vi "LVUSBRH2_Measurement_main.vi"() -> ()   [LabVIEW 2020]
uses:
  <vilib>/Utility/sysdir.llb/System Directory Type.ctl
  <vilib>/Utility/miscctls.llb/LVPointTypeDef.ctl
  <vilib>/Instr/_visa.llb/VISA Flush IO Buffer Mask.ctl
  <vilib>/Platform/browser.llb/Open URL in Default Browser (string).vi
  <vilib>/Instr/_visa.llb/VISA Configure Serial Port (Instr).vi
  <vilib>/ptbypt/NI_PtbyPt.lvlib
panel:
  in  "USBRH Link":bool caption="USBRRH2 link:"
  out "title":string="LVUSBRH2 Measure"
  out "Measure":bool
  in  "Btn Exit":bool
  in  "LED 2":bool
  in  "LED 1":bool
  in  "Btn Settings":bool
  in  "Btn Stop":bool
  in  "Btn Start":bool
  out "Humid":dbl caption="RHumidity(%)" format="%.2f"
  out "Temp":dbl caption="Temperature(C)" format="%.2f"
  out "chart 1":cluster{dbl, dbl}(graph)
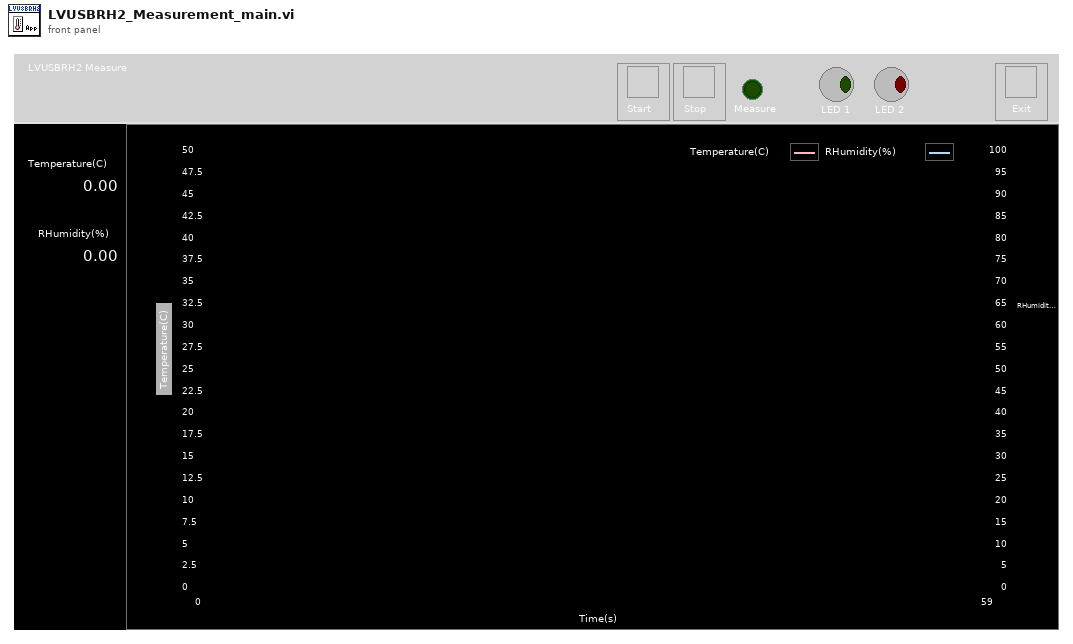
[diagram p1: front panel]
types:
  T1 = typedef "System Directory Type.ctl" = i32
  T2 = typedef "LVPointTypeDef.ctl" = cluster{"Horizontal":i16, "Vertical":i16}
  T3 = cluster{bool, "include Ctrl key?":bool, string}[]
  T4 = cluster{"配列[0]":i16, "配列[1]":i16, "配列[2]":i16, "配列[3]":i16}
  T5 = typedef "VISA Flush IO Buffer Mask.ctl" = u16
  T6 = typedef "LVRectTypeDef.ctl" = cluster{"left":i16, "top":i16, "right":i16, "bottom":i16}
  T7 = enum32{"invalid app kind", "Development System", "Run Time System", "Student Edition", "Embedded LabVIEW", "Evaluation", "Custom"}
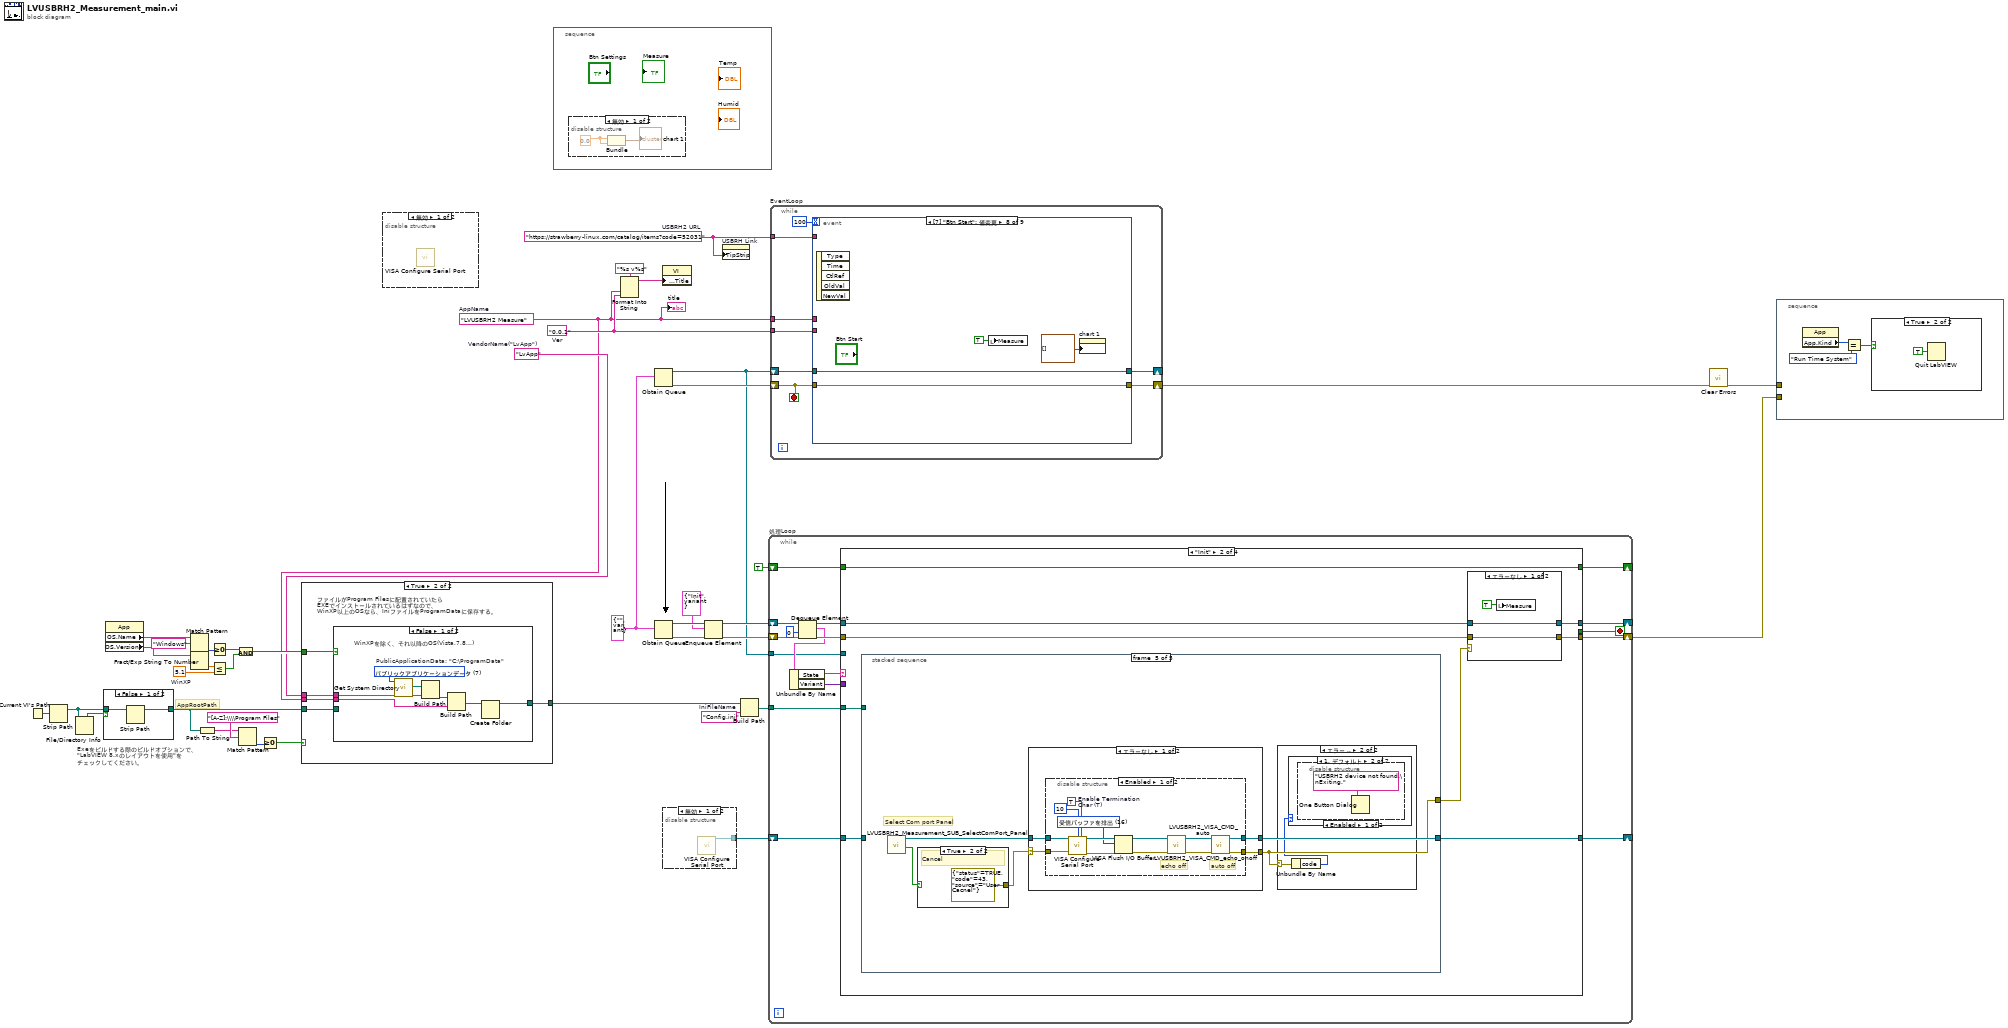
[diagram p0: block diagram]
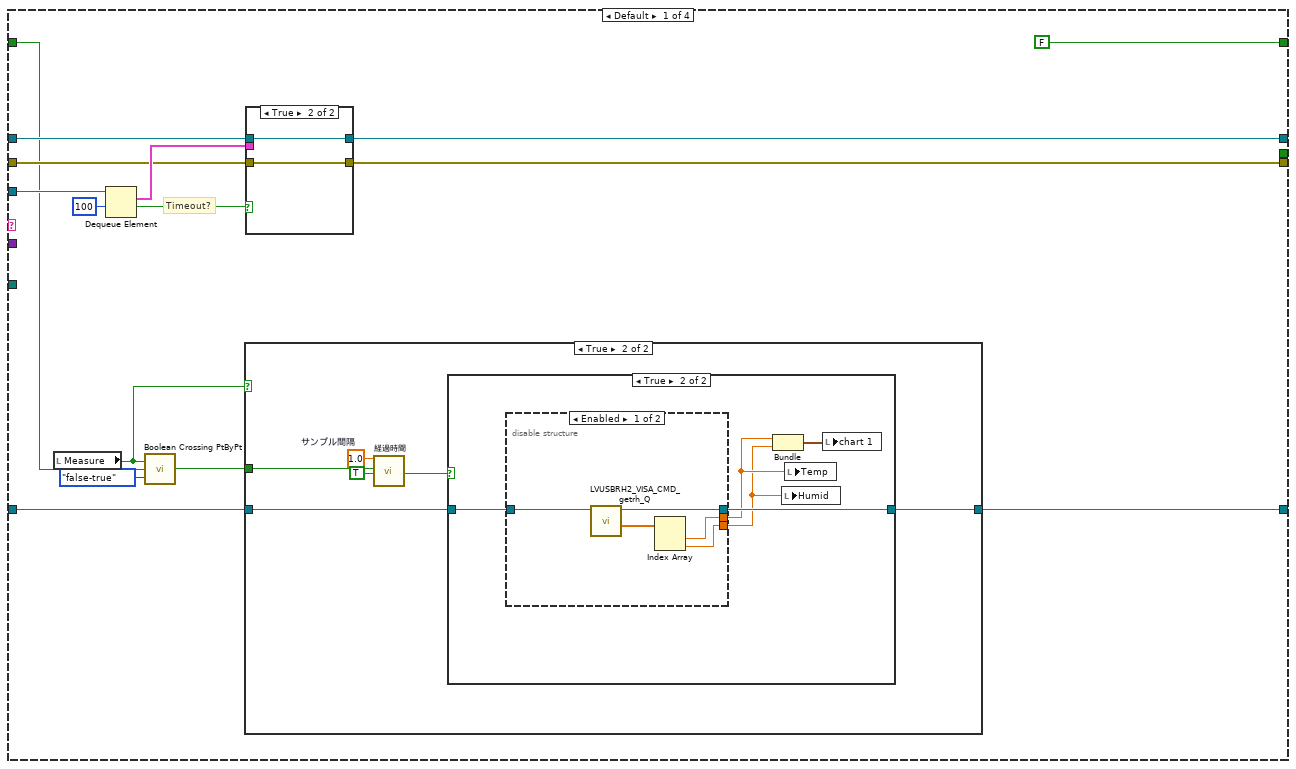
[diagram p9: hidden frame]
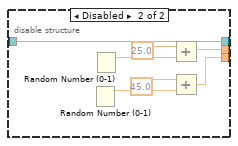
[diagram p12: hidden frame]
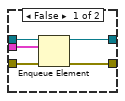
[diagram p13: hidden frame]
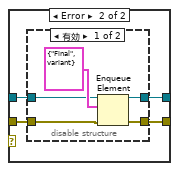
[diagram p14: hidden frame]
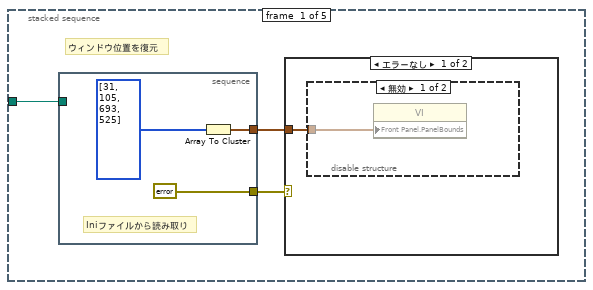
[diagram p16: hidden frame]
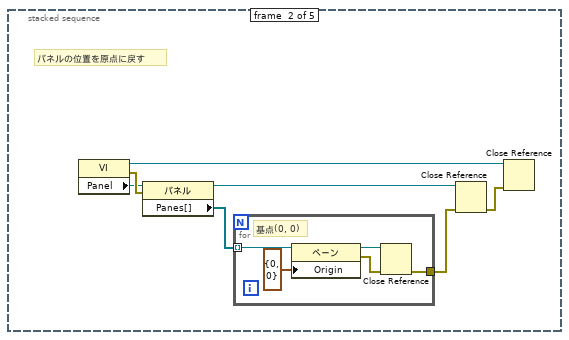
[diagram p19: hidden frame]
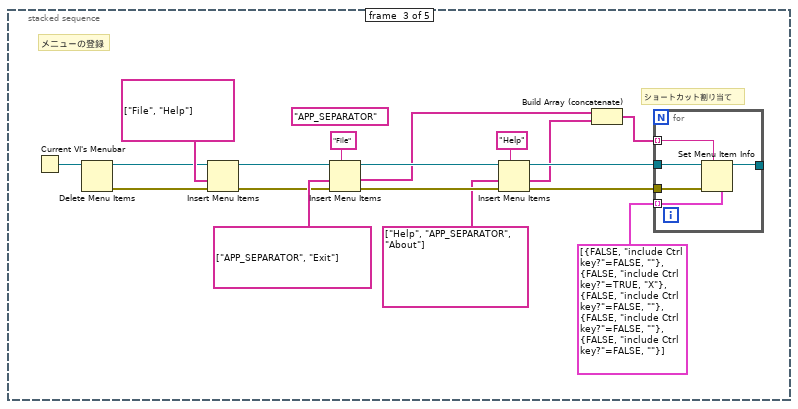
[diagram p20: hidden frame]
diagram:
  w3 = "LvApp"  # VendorName("LvApp")
  w17 = 5.1  # WinXP
  w23 = "https://strawberry-linux.com/catalog/items?code=52031"  # USBRH2 URL
  w25 = "Config.ini"  # IniFileName
  w28 = "0.0.1"  # Ver
  w2 = "LVUSBRH2 Measure"  # AppName
  w39 = cluster{"State":string, "Variant":variant} {"State"="", "Variant"=variant}
  # "Exeをビルドする際のビルドオプションで、\n\"LabVIEW 8.xのレイアウトを使用\"を\nチェックしてください。"
  # "AppRootPath"
  n1 = Current VI's Path() -> (path=w11:path)
  n2 = Strip Path(path=w11) -> (stripped path=w12:path)  [unwired: 1 out]
  n3 = File/Directory Info(path=w12) -> (directory=w13:bool)  [unwired: 1 in, 6 out]
  n4 = case shown="FALSE" w13 {
    tunnel: w12 -> [w41 w42]
    tunnel: [w40 w42] -> w8
    frame False {
      n5 = Strip Path(path=w41) -> (stripped path=w40:path)  [unwired: 1 out]
    }
    frame True {
    }
  }
  n6 = property class="App"() -> ("OS.Name"=w21:string, "OS.Version"=w19:string)  [unwired: 2 in, 2 out]
  n7 = Match Pattern(string=w21, regular expression="Windows" ("正規表現")) -> (offset past match=w16:i32)  [unwired: 1 in, 3 out]
  n8 = Fract/Exp String To Number(string=w19) -> (number=w18:dbl)  [unwired: 3 in, 1 out]
  n9 = Path To String(path=w8) -> (string=w7:string)
  n10 = Greater Or Equal To 0?(x=w16) -> (x >= 0?=w15:bool)
  n11 = Less Or Equal?(x=w18, y=w17) -> (x <= y?=w14:bool)
  n12 = And(x=w15, y=w14) -> (x .and. y?=w10:bool)
  n13 = Match Pattern(string=w7, regular expression="[A-Z]:\\\\Program Files" ("正規表現")) -> (offset past match=w6:i32)  [unwired: 1 in, 3 out]
  n14 = Greater Or Equal To 0?(x=w6) -> (x >= 0?=w5:bool)
  n15 = case shown="TRUE" w5 {
    tunnel: w2 -> [_ w48]
    tunnel: [w43 w46] -> w4
    tunnel: w3 -> [_ w47]
    tunnel: w10 -> [_ w45]
    tunnel: w8 -> [w43 w44]
    frame False {
      # "ファイルがProgram Filesに配置されていなかったら\n開発システムでソースから実行しているか、\nExeで適当なフォルダから実行されているので、\nIniファイルは、EXE, またはTop VI と同じ場所に保存"
    }
    frame True {
      # "ファイルがProgram Filesに配置されていたら\nEXEでインストールされているはずなので、\nWinXP以上のOSなら、IniファイルをProgramDataに保存する。"
      n16 = case shown="FALSE" w45 {
        tunnel: w48 -> [w52 _]
        tunnel: w47 -> [w50 _]
        tunnel: [w49 w56] -> w46
        tunnel: w44 -> [_ w56]
        frame False {
          w55 = T1 7 items=["ユーザホーム"=0, "ユーザデスクトップ"=1, "ユーザドキュメント"=2, "ユーザアプリケーションデータ"=3, "ユーザ設定"=4, "ユーザ一時"=5, "パブリックドキュメント"=6, "パブリックアプリケーションデータ"=7, "パブリック環境設定"=8, "パブリックキャッシュ"=13, "システムコアライブラリ"=9, "システムインストールされたライブラリ"=10, "アプリケーションファイル"=11, "ブート容量ルート"=12] ("system directory type")
          # "PublicApplicationData: \"C:\\ProgramData\""
          # "WinXPを除く、それ以降のOS(Vista,7,8,..)"
          n17 = call <vilib>:"Get System Directory.vi"("system directory type"=w55) -> ("system directory"=w54:path)  [unwired: 10 in]
          n18 = Build Path(base path=w54, name or relative path=w50) -> (appended path=w53:path)
          n19 = Build Path(base path=w53, name or relative path=w52) -> (appended path=w51:path)
          n20 = Create Folder(path (use dialog)=w51) -> (created path=w49:path)  [unwired: 2 in, 2 out]
        }
        frame True {
        }
      }
    }
  }
  n21 = disable-structure shown="無効" {
    frame Disabled {
      n22 = call-poly "VISA Configure Serial Port"() -> ()  [unwired: 14 in, 2 out]
    }
    frame Enabled {
    }
  }
  n23 = stacked-sequence {
    frame #0 {
      n24 = disable-structure shown="無効" {
        frame Disabled {
          w58 = 0.0
          n25 = Bundle(w58, w58) -> (→"chart 1":cluster{dbl, dbl})  [unwired: 1 in]
        }
        frame Enabled {
        }
      }
    }
  }
  n26 = Format Into String(format string="%s v%s" ("形式文字列"), w2, w28) -> (resulting string=w26:string)  [unwired: 2 in, 1 out]
  n27 = Obtain Queue(element data type=w39) -> (queue out=w32:refnum<queue>, error out=w38:errorcluster)  [unwired: 4 in, 1 out]
  n28 = Obtain Queue(element data type=w39) -> (queue out=w37:refnum<queue>, error out=w35:errorcluster)  [unwired: 4 in, 1 out]
  n29 = property class="VI"("Front Panel.Title"=w26) -> ()  [unwired: 2 in, 2 out]
  n30 = disable-structure shown="無効" {
    disable-tunnel: [w59 _] -> w1
    frame Disabled {
      n31 = call-poly "VISA Configure Serial Port"() -> ("VISA resource name out"=w59:refnum<visa-resource-name>)  [unwired: 14 in, 1 out]
    }
    frame Enabled {
    }
  }
  n32 = Enqueue Element(queue=w37, element=cluster{"State":string, "Variant":variant} {"State"="Init", "Variant"=variant}, error in (no error)=w35) -> (queue out=w36:refnum<queue>, error out=w34:errorcluster)  [unwired: 1 in, 1 out]
  n33 = property on="USBRH Link" class="Bool"("TipStrip"=w23) -> ()  [unwired: 2 in, 2 out]
  n34 = Build Path(base path=w4, name or relative path=w25) -> (appended path=w29:path)
  n35 = while "処理Loop" {
    shift-right: [w71] -> _
    shift-left: w36 -> [w76]
    shift-right: [w70] -> w22
    shift-left: w34 -> [w73]
    tunnel: w32 -> [w66]
    tunnel: w29 -> [w64]
    shift-right: [w63] -> _
    shift-left: w1 -> [w62]
    shift-right: [w60] -> _
    shift-left: TRUE -> [w61]
    stop <- w65 stop-if-true
    n36 = Dequeue Element(queue=w76, timeout in ms (-1)=0 ("タイムアウト（ms）（-1）"), error in (no error)=w73) -> (queue out=w75:refnum<queue>, element=w69:cluster{"State":string, "Variant":variant}, error out=w72:errorcluster)  [unwired: 1 out]
    n37 = Unbundle By Name(w69) -> ("State"=w68:string, "Variant"=w67:variant)
    n38 = case shown="\"Init\"" w68 {
      selector: w68 -> [_ _ _ w245]
      tunnel: w75 -> [w88 w129 w233 w247]
      tunnel: w66 -> [w91 _ w231 _]
      tunnel: w72 -> [w86 w128 w230 w246]
      tunnel: [w87 w127 refnum<queue> refnum ("queue out") w247] -> w71
      tunnel: [w85 w126 w229 w246] -> w70
      tunnel: w67 -> [_ _ _ w244]
      tunnel: [_ _ TRUE _] -> w65
      tunnel: w64 -> [_ w132 w228 _]
      tunnel: [w82 w131 refnum<visa-resource-name> refnum ("VISA resource name out") w241] -> w63
      tunnel: w62 -> [w84 w124 w226 w240]
      tunnel: w61 -> [w80 w125 w227 w242]
      tunnel: [FALSE w125 w227 w242] -> w60
      frame Default {
        # "Timeout?"
        n39 = local read "Measure"() -> (w78:bool)
        n40 = Dequeue Element(queue=w91, timeout in ms (-1)=100 ("タイムアウト（ms）（-1）")) -> (element=w89:cluster{"State":string, "Variant":variant}, timed out?=w83:bool)  [unwired: 1 in, 2 out]
        n41 = call <vilib>:"Boolean Crossing PtByPt.vi"("initialize"=w80, "direction"=enum16{"either", "false-true", "true-false"}."false-true", "input"=w78) -> ("crossing"=w77:bool)
        n42 = case shown="TRUE" w78 {
          tunnel: w84 -> [w92 w94]
          tunnel: [w92 w93] -> w82
          tunnel: w77 -> [_ w96]
          frame False {
          }
          frame True {
            w97 = 1.0  # サンプル間隔
            n43 = call "経過時間"("Time Target (s)"=w97, "Reset"=w96, "Auto Reset"=TRUE) -> ("Time has Elapsed"=w95:bool)  [unwired: 9 in, 7 out]
            n44 = case shown="TRUE" w95 {
              tunnel: w94 -> [w99 w103]
              tunnel: [w99 w102] -> w93
              frame False {
              }
              frame True {
                n45 = disable-structure shown="Enabled" {
                  disable-tunnel: w103 -> [w109 w116]
                  disable-tunnel: [w108 w116] -> w102
                  disable-tunnel: [w106 w115] -> w101
                  disable-tunnel: [w105 w113] -> w100
                  frame Enabled {
                    n46 = call "LVUSBRH2_VISA_CMD_getrh_Q.vi"("VISA rssc"=w109) -> ("data[]"=w107:dbl[], "VISA rssc out"=w108:refnum<visa-resource-name>)  [unwired: 8 in, 1 out]
                    n47 = Index Array(array=w107) -> (element #1=w106:dbl, element #2=w105:dbl)  [unwired: 2 in]
                  }
                  frame Disabled {
                    n48 = Random Number (0-1)() -> (number: 0 to 1=w110:dbl)
                    n49 = Random Number (0-1)() -> (number: 0 to 1=w111:dbl)
                    n50 = Add(x=25.0, y=w111) -> (x+y=w115:dbl)
                    n51 = Add(x=45.0, y=w110) -> (x+y=w113:dbl)
                  }
                }
                n52 = Bundle(w101, w100) -> (w104:cluster{dbl, dbl})  [unwired: 1 in]
                n53 = local write "Humid"(w100) -> ()
                n54 = local write "Temp"(w101) -> ()
                n55 = local write "chart 1"(w104) -> ()
              }
            }
          }
        }
        n56 = case shown="TRUE" w83 {
          tunnel: w89 -> [w121 _]
          tunnel: w88 -> [w120 w123]
          tunnel: [w119 w123] -> w87
          tunnel: w86 -> [w118 w122]
          tunnel: [w117 w122] -> w85
          frame False {
            n57 = Enqueue Element(queue=w120, element=w121, error in (no error)=w118) -> (queue out=w119:refnum<queue>, error out=w117:errorcluster)  [unwired: 1 in, 1 out]
          }
          frame True {
          }
        }
      }
      frame "Init" {
        n58 = stacked-sequence {
          tunnel: w132 -> [w147 _ _ _ _]
          tunnel: [_ _ _ _ w199] -> w131
          tunnel: [_ _ _ _ w195] -> w130
          tunnel: w124 -> [_ _ _ _ _]
          frame #0 {
            # "ウィンドウ位置を復元"
            n59 = stacked-sequence {
              tunnel: [w150] -> w149
              tunnel: [errorcluster {"status"=FALSE, "code"=0, "source"=""} ("error in (no error)")] -> w148
              tunnel: w147 -> [_]
              frame #0 {
                # "Iniファイルから読み取り"
                n60 = Array To Cluster(array=i16[] [31, 105, 693, 525] ("配列")) -> (cluster=w150:T4)
              }
            }
            n61 = case shown="エラーなし" w148 {
              tunnel: w149 -> [w153 _]
              frame No Error {
                n62 = disable-structure shown="無効" {
                  disable-tunnel: w153 -> [w154 _]
                  frame Disabled {
                    n63 = property class="VI"("Front Panel.PanelBounds"=w154) -> ()  [unwired: 2 in, 2 out]
                  }
                  frame Enabled {
                  }
                }
              }
              frame Error {
              }
            }
          }
          frame #1 {
            # "パネルの位置を原点に戻す"
            n64 = property class="VI"() -> (reference out=w158:refnum<vi>, error out=w161:errorcluster, "Panel"=w155:refnum<vi>)  [unwired: 2 in]
            n65 = property on="プロパティノード" class="パネル"(reference=w155, error in=w161) -> (reference out=w157:refnum<vi>, "Panes[]"=w156:refnum<vi>[])  [unwired: 1 out]
            n66 = for {
              tunnel: w156 -> [w166] mode=indexing
              tunnel: [w163] -> w159
              # "基点(0, 0)"
              n67 = property on="プロパティノード" class="ペーン"(reference=w166, "Origin"=T2 {"Horizontal"=0, "Vertical"=0} ("原点")) -> (reference out=w165:refnum<vi>, error out=w164:errorcluster)  [unwired: 1 in]
              n68 = Close Reference(reference=w165, error in (no error)=w164) -> (error out=w163:errorcluster)
            }
            n69 = Close Reference(reference=w157, error in (no error)=w159) -> (error out=w160:errorcluster)
            n70 = Close Reference(reference=w158, error in (no error)=w160) -> ()  [unwired: 1 out]
          }
          frame #2 {
            (unwired) "APP_SEPARATOR"
            # "ショートカット割り当て"
            # "メニューの登録"
            n71 = Current VI's Menubar() -> (w175:refnum<k9>)
            n72 = Delete Menu Items(9:w175) -> (0:w177:errorcluster, 3:w176:refnum<k9>)  [unwired: 3 in]
            n73 = Insert Menu Items(6:w177, 7:string[] ["File", "Help"] ("item tags"), 9:w176) -> (0:w181:errorcluster, 3:w180:refnum<k9>)  [unwired: 3 in, 1 out]
            n74 = Insert Menu Items(5:"File" ("menu tag"), 6:w181, 7:string[] ["APP_SEPARATOR", "Exit"] ("item tags"), 9:w180) -> (0:w184:errorcluster, 1:w170:string[], 3:w183:refnum<k9>)  [unwired: 2 in]
            n75 = Insert Menu Items(5:"Help" ("menu tag"), 6:w184, 7:string[] ["Help", "APP_SEPARATOR", "About"] ("item tags"), 9:w183) -> (0:w171:errorcluster, 1:w169:string[], 3:w172:refnum<k9>)  [unwired: 2 in]
            n76 = Build Array (concatenate)(w170, w169) -> (w167:string[])
            n77 = for {
              tunnel: w172 -> [w189]
              tunnel: w171 -> [w188]
              tunnel: [w187] -> _
              tunnel: T3 [{FALSE, "include Ctrl key?"=FALSE, ""}, {FALSE, "include Ctrl key?"=TRUE, "X"}, {FALSE, "include Ctrl key?"=FALSE, ""}, {FALSE, "include Ctrl key?"=FALSE, ""}, {FALSE, "include Ctrl key?"=FALSE, ""}] -> [w186] mode=indexing
              tunnel: w167 -> [w185] mode=indexing
              n78 = Set Menu Item Info(4:w186, 7:w185, 8:w188, 11:w189) -> (3:w187:refnum<k9>)  [unwired: 3 in, 1 out]
            }
          }
          frame #3 {
            w190 = 0.0 ("Temp")
            # "パネル制御器の初期化"
            n79 = local write "Measure"(FALSE ("Measure")) -> ()
            n80 = property on="chart 1" class="WFChart (指定)"("History Data"=cluster{dbl, dbl}[] [] ("履歴データ")) -> ()  [unwired: 2 in, 2 out]
            n81 = property on="LED 1" class="Bool (指定)"("TipStrip"="Turn on/off LED1 on USBRH2" ("ヒントラベル")) -> ()  [unwired: 2 in, 2 out]
            n82 = property on="LED 2" class="Bool (指定)"("TipStrip"="Turn on/off LED2 on USBRH2" ("ヒントラベル")) -> ()  [unwired: 2 in, 2 out]
            n83 = local write "Humid"(w190) -> ()
            n84 = local write "Temp"(w190) -> ()
          }
          frame #4 {
            # "Select Com port Panel"
            n85 = call "LVUSBRH2_Measurement_SUB_SelectComPort_Panel.vi"() -> ("Cancel?"=w197:bool, "VISA rsrc out"=w198:refnum<visa-resource-name>)  [unwired: 10 in]
            n86 = case shown="TRUE" w197 {
              tunnel: [_ errorcluster {"status"=TRUE, "code"=43, "source"="User Cacnel"} ("エラー定数")] -> w196
              frame False {
              }
              frame True {
                # "Cancel"
              }
            }
            n87 = case shown="エラーなし" w196 {
              selector: w196 -> [w206 w223]
              tunnel: w198 -> [w207 w224]
              tunnel: [w204 w224] -> w199
              tunnel: [w205 w223] -> w195
              frame No Error {
                n88 = disable-structure shown="Enabled" {
                  disable-tunnel: w207 -> [w220 w222]
                  disable-tunnel: w206 -> [w219 w221]
                  disable-tunnel: [w215 w221] -> w205
                  disable-tunnel: [w214 w222] -> w204
                  frame Enabled {
                    w208 = TRUE  # Enable Termination Char (T)
                    w212 = T5 16 items=["受信バッファを排出"=16, "送信バッファをデバイスに書き込む"=32, "受信バッファを排出 (I/Oなし)"=64, "送信バッファを排出"=128] ("Mask")
                    # "auto off"
                    # "echo off"
                    n89 = call-poly "VISA Configure Serial Port"("VISA resource name"=w220, "termination char\n(0xA = '\\n' = LF)"=u8 10 ("termination char\n(0xA = '\\n' = LF)"), "Enable Termination\nChar (T)"=w208, "error in (no error)"=w219) -> ("VISA resource name out"=w218:refnum<visa-resource-name>, "error out"=w211:errorcluster)  [unwired: 10 in]
                    n90 = VISA Flush I/O Buffer(VISA resource name=w218, mask (16)=w212, error in (no error)=w211) -> (VISA resource name out=w213:refnum<visa-resource-name>, error out=w210:errorcluster)
                    n91 = call "LVUSBRH2_VISA_CMD_echo_onoff.vi"("error in (no error)"=w210, "VISA rssc"=w213) -> ("error out"=w216:errorcluster, "VISA rssc out"=w217:refnum<visa-resource-name>)  [unwired: 8 in]
                    n92 = call "LVUSBRH2_VISA_CMD_auto.vi"("error in (no error)"=w216, "VISA rssc"=w217) -> ("error out"=w215:errorcluster, "VISA rssc out"=w214:refnum<visa-resource-name>)  [unwired: 8 in]
                  }
                  frame Disabled {
                  }
                }
              }
              frame Error {
              }
            }
            n93 = case shown="エラー .." w195 {
              selector: w195 -> [_ w201]
              frame No Error {
              }
              frame Error {
                n94 = Unbundle By Name(w201) -> ("code"=w200:i32)
                n95 = case shown="1, デフォルト" w200 {
                  frame 43 {
                  }
                  frame 1, Default {
                    n96 = disable-structure shown="Enabled" {
                      frame Enabled {
                        n97 = One Button Dialog(message="USBRH2 device not found.\nExiting." ("メッセージ")) -> ()  [unwired: 1 in, 1 out]
                      }
                      frame Disabled {
                      }
                    }
                  }
                }
              }
            }
          }
        }
        n98 = case shown="エラーなし" w130 {
          tunnel: w129 -> [w135 w139]
          tunnel: w128 -> [w134 w137]
          tunnel: [w135 w138] -> w127
          tunnel: [w134 w136] -> w126
          frame No Error {
            n99 = local write "Measure"(TRUE ("Measure")) -> ()
          }
          frame Error {
            n100 = disable-structure shown="有効" {
              disable-tunnel: w139 -> [w143 w146]
              disable-tunnel: [w142 w146] -> w138
              disable-tunnel: w137 -> [w141 w145]
              disable-tunnel: [w140 w145] -> w136
              frame Enabled {
                n101 = Enqueue Element(queue=w143, element=cluster{string, "バリアント":variant} {"Final", "バリアント"=variant}, error in (no error)=w141) -> (queue out=w142:refnum<queue>, error out=w140:errorcluster)  [unwired: 1 in, 1 out]
              }
              frame Disabled {
              }
            }
          }
        }
      }
      frame "Final" {
        n102 = stacked-sequence {
          tunnel: w228 -> [w236]
          frame #0 {
            n103 = property class="VI"() -> ("Front Panel.PanelBounds"=w235:T6)  [unwired: 2 in, 2 out]
            n104 = stacked-sequence {
              tunnel: w236 -> [_]
              tunnel: w235 -> [w237]
              frame #0 {
                n105 = Cluster To Array(cluster=w237) -> ()  [unwired: 1 out]
              }
            }
          }
        }
        n106 = Release Queue(queue=w233, error in (no error)=w230) -> (error out=w229:errorcluster)  [unwired: 1 in, 2 out]
        n107 = Release Queue(queue=w231) -> ()  [unwired: 2 in, 3 out]
        n108 = VISA Close(VISA resource name=w226) -> ()  [unwired: 1 in, 1 out]
      }
      frame "LED 1", "LED 2" {
        n109 = Variant To Data(type=TRUE, Variant=w244) -> (data=w238:bool)  [unwired: 1 in, 1 out]
        n110 = case shown="\"LED 1\", デフォルト" w245 {
          tunnel: [1 2] -> w239
          frame "LED 1", Default {
          }
          frame "LED 2" {
          }
        }
        n111 = call "LVUSBRH2_VISA_CMD_led_onoff.vi"("Sw"=w238, "CH#(1)"=w239, "VISA rssc"=w240) -> ("VISA rssc out"=w241:refnum<visa-resource-name>)  [unwired: 7 in, 1 out]
      }
    }
  }
  n112 = while "EventLoop" {
    shift-right: [w255] -> _
    shift-left: w32 -> [w256]
    shift-right: [w254] -> w31
    shift-left: w38 -> [w253]
    tunnel: w2 -> [w252]
    tunnel: w28 -> [w251]
    tunnel: w23 -> [w250]
    stop <- w253 stop-if-true
    n113 = event shown="[7] \"Btn Start\": 値変更" {
      selector: _ -> [_ _ _ _ _ _ _ _ _]
      dyn-events: _ -> [_ _ _ _ _ _ _ _ _]
      timeout: 100 -> [_ _ _ _ _ _ _ _ _]
      tunnel: w256 -> [w261 w267 w273 w281 w299 w304 w312 w317 w320]
      tunnel: [w258 w266 w272 w280 w299 w303 w311 w317 w320] -> w255
      tunnel: w253 -> [w260 w265 w271 w279 w298 w302 w310 w316 w319]
      tunnel: [w259 w264 w270 w278 w298 w301 w309 w316 w319] -> w254
      tunnel: w252 -> [_ _ _ w276 _ _ _ _ _]
      tunnel: w251 -> [_ _ _ w275 _ _ _ _ _]
      tunnel: w250 -> [_ _ _ _ w297 _ _ _ _]
      event Timeout {
        n114 = event-data() -> ()  [unwired: 1 in, 2 out]
        n115 = Get Queue Status(queue=w261, error in (no error)=w260) -> (queue out=w258:refnum<queue>, error out=w259:errorcluster)  [unwired: 1 in, 6 out]
      }
      event Application Instance Close? {
        n116 = event-data() -> ()  [unwired: 1 in, 4 out]
        n117 = Enqueue Element(queue=w267, element=cluster{string, "バリアント":variant} {"Final", "バリアント"=variant}, error in (no error)=w265) -> (queue out=w266:refnum<queue>, error out=w264:errorcluster)  [unwired: 1 in, 1 out]
        n118 = event-data("SilentShutdown"=TRUE, "Discard?"=FALSE ("破棄?")) -> ()  [unwired: 1 in, 1 out]
      }
      event Panel Close? {
        n119 = event-data() -> ()  [unwired: 1 in, 3 out]
        n120 = Enqueue Element(queue=w273, element=cluster{string, "バリアント":variant} {"Final", "バリアント"=variant}, error in (no error)=w271) -> (queue out=w272:refnum<queue>, error out=w270:errorcluster)  [unwired: 1 in, 1 out]
        n121 = event-data("Discard?"=TRUE) -> ()  [unwired: 1 in, 1 out]
      }
      event Menu Selection (User) {
        n122 = event-data() -> ("ItemPath"=w277:string)  [unwired: 1 in, 5 out]
        n123 = case shown="\"File:Exit\"" w277 {
          tunnel: w281 -> [w283 w288 w294 w296]
          tunnel: [w283 w287 w294 w296] -> w280
          tunnel: w279 -> [w282 w286 w293 w295]
          tunnel: [w282 w285 w293 w295] -> w278
          tunnel: w276 -> [_ _ w292 _]
          tunnel: w275 -> [_ _ w291 _]
          frame Default {
          }
          frame "File:Exit" {
            n124 = Enqueue Element(queue=w288, element=cluster{string, "バリアント":variant} {"Final", "バリアント"=variant}, error in (no error)=w286) -> (queue out=w287:refnum<queue>, error out=w285:errorcluster)  [unwired: 1 in, 1 out]
          }
          frame "Help:About" {
            n125 = Format Into String(format string="%s\n\nVersion : %s" ("メッセージ"), w292, w291) -> (resulting string=w289:string)  [unwired: 2 in, 1 out]
            n126 = One Button Dialog(message=w289) -> ()  [unwired: 1 in, 1 out]
          }
          frame "Help:Help" {
          }
        }
      }
      event "USBRH Link": Value Change {
        n127 = event-data() -> ()  [unwired: 1 in, 5 out]
        n128 = call-poly <vilib>:"Open URL in Default Browser.vi"("URL"=w297) -> ()  [unwired: 5 in, 2 out]
      }
      event "Btn Exit": Value Change {
        n129 = event-data() -> ()  [unwired: 1 in, 5 out]
        n130 = Enqueue Element(queue=w304, element=cluster{string, "バリアント":variant} {"Final", "バリアント"=variant}, error in (no error)=w302) -> (queue out=w303:refnum<queue>, error out=w301:errorcluster)  [unwired: 1 in, 1 out]
      }
      event "LED 1", "LED 2": Value Change {
        n131 = event-data() -> ("CtlRef"=w313:refnum<vi>, "NewVal"=w305:bool)  [unwired: 1 in, 3 out]
        n132 = property class="Bool (指定)"(reference=w313) -> ("Label.Text"=w306:string)  [unwired: 1 in, 2 out]
        n133 = Bundle By Name(cluster=cluster{"State":string, "Variant":variant} {"State"="", "Variant"=variant}, "State"=w306, "Variant"=w305) -> (w307:cluster{"State":string, "Variant":variant})
        n134 = Enqueue Element(queue=w312, element=w307, error in (no error)=w310) -> (queue out=w311:refnum<queue>, error out=w309:errorcluster)  [unwired: 1 in, 1 out]
      }
      event "Btn Start": Value Change {
        n135 = event-data() -> ()  [unwired: 1 in, 5 out]
        n136 = local write "Measure"(TRUE ("Measure")) -> ()
        n137 = property on="chart 1" class="WFChart (指定)"("History Data"=cluster{dbl, dbl}[] [] ("履歴データ")) -> ()  [unwired: 2 in, 2 out]
      }
      event "Btn Stop": Value Change {
        n138 = event-data() -> ()  [unwired: 1 in, 5 out]
        n139 = local write "Measure"(FALSE ("Measure")) -> ()
      }
    }
  }
  n140 = call <vilib>:"Clear Errors.vi"("error in (no error)"=w31) -> ("error out"=w30:errorcluster)  [unwired: 5 in, 1 out]
  n141 = stacked-sequence {
    tunnel: w30 -> [_]
    tunnel: w22 -> [_]
    frame #0 {
      n142 = property class="App"() -> ("App.Kind"=w323:T7)  [unwired: 2 in, 2 out]
      n143 = Equal?(x=w323, y=T7."Run Time System" ("アプリケーション:種類")) -> (x = y?=w321:bool)
      n144 = case shown="TRUE" w321 {
        frame False {
        }
        frame True {
          n145 = Quit LabVIEW(quit? (T)=TRUE ("終了?（T）")) -> ()
        }
      }
    }
  }
  "title" <- w2
